vi "Control Simu.vi"(6 "Error Feedback":bool, 7 "Watchdog Feedback In":i32, 10 "Error Ch":bool[](array[boolean]), 11 "Controls In":T1) -> (3 "Controls Out":T2, 4 "Error Feedback out":bool, 5 "Watchdog Feedback Out":i32)   [LabVIEW 2024]
uses:
  Capabilities/Capabilities/High Level Capabilities/Cycler Cluster/Producer Control.ctl
  Capabilities/Capabilities/High Level Capabilities/Cycler Cluster/Cycler Cluster.lvclass
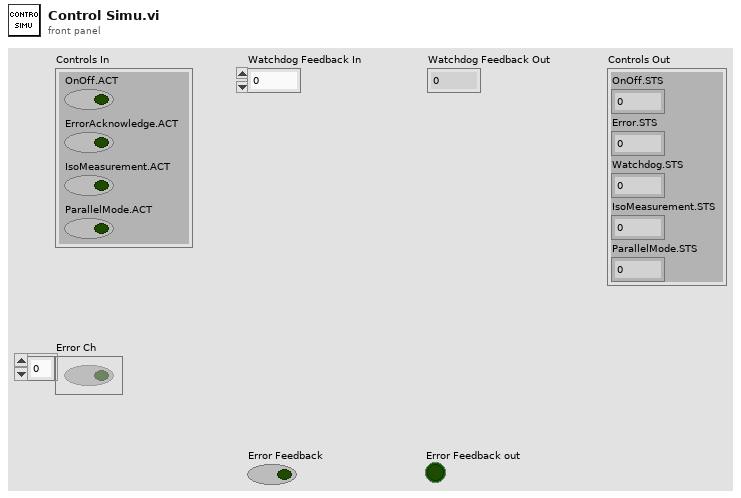
[diagram p1: front panel]
types:
  T1 = cluster{"OnOff.ACT":bool, "ErrorAcknowledge.ACT":bool, "IsoMeasurement.ACT":bool, "ParallelMode.ACT":bool}
  T2 = typedef "Cycler Cluster.lvclass/Producer Control.ctl" = cluster{"OnOff.STS":i32, "Error.STS":i32, "Watchdog.STS":i32, "IsoMeasurement.STS":i32, "ParallelMode.STS":i32}
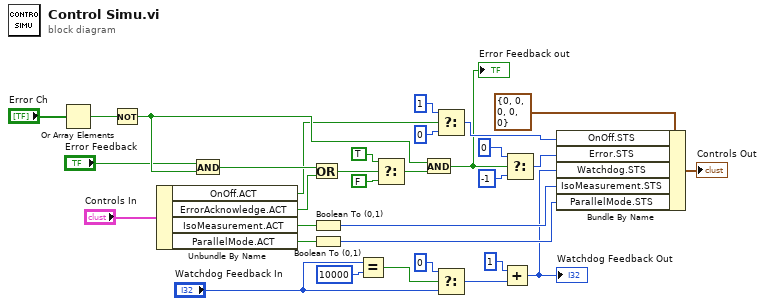
[diagram p0: block diagram]
diagram:
  n1 = Or Array Elements(Boolean array="Error Ch") -> (logical OR=w26:bool)
  n2 = Not(x=w26) -> (.not. x?=w29:bool)
  n3 = Unbundle By Name("Controls In") -> ("OnOff.ACT"=w15:bool, "ErrorAcknowledge.ACT"=w14:bool, "IsoMeasurement.ACT"=w13:bool, "ParallelMode.ACT"=w12:bool)
  n4 = And(x="Error Feedback", y=w29) -> (x .and. y?=w30:bool)
  n5 = Or(x=w30, y=w14) -> (x .or. y?=w27:bool)
  n6 = Boolean To (0,1)(Boolean=w13) -> (0, 1=w9:i16)
  n7 = Boolean To (0,1)(Boolean=w12) -> (0, 1=w10:i16)
  n8 = Equal?(x="Watchdog Feedback In", y=10000) -> (x = y?=w31:bool)
  n9 = Select(t=TRUE, s=w27, f=FALSE) -> (s? t:f=w28:bool)
  n10 = And(x=w29, y=w28) -> (x .and. y?=w2:bool)
  "Error Feedback out" <- w2
  n11 = Select(t=1, s=w15, f=0) -> (s? t:f=w7:i32)
  n12 = Select(t=0, s=w31, f="Watchdog Feedback In") -> (s? t:f=w32:i32)
  n13 = Add(x=1, y=w32) -> (x+y=w3:i32)
  "Watchdog Feedback Out" <- w3
  n14 = Select(t=0, s=w2, f=-1) -> (s? t:f=w8:i32)
  n15 = Bundle By Name(cluster=T2 {"OnOff.STS"=0, "Error.STS"=0, "Watchdog.STS"=0, "IsoMeasurement.STS"=0, "ParallelMode.STS"=0} ("Producer Control"), "OnOff.STS"=w7, "Error.STS"=w8, "Watchdog.STS"=w3, "IsoMeasurement.STS"=w9, "ParallelMode.STS"=w10) -> (→"Controls Out":T2)
